vi "Calculate Throughput Wrapper.vi"(4 "transfers":u64, 5 "iterations":u64) -> (1 "throughput (B/s)":dbl)   [LabVIEW 2013]
doc: "This SubVI collects and feeds Data to the \"Calculate Throutput\" SubVI."
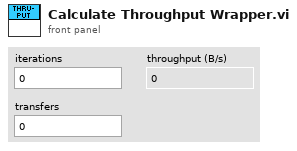
[diagram p1: front panel]
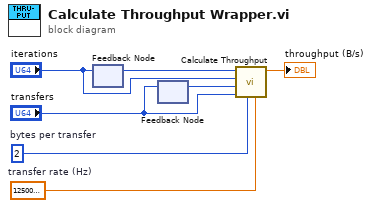
[diagram p0: block diagram]
diagram:
  w6 = 125000000.0  # transfer rate (Hz)
  w5 = u64 2  # bytes per transfer
  n1 = feedback #1() -> (w3:u64)  [unwired: 1 in]
  n2 = feedback-in #1("iterations") -> ()
  n3 = feedback #2() -> (w4:u64)  [unwired: 1 in]
  n4 = feedback-in #2("transfers") -> ()
  n5 = call "Calculate Throughput.vi"("FPGA FIFO clock"=w6, "bytes per element"=w5, "transfer count"="transfers", "previous transfer count"=w4, "iteration count"="iterations", "previous iteration count"=w3) -> ("throughput (B/s)"=→"throughput (B/s)":dbl)  [unwired: 5 in]
